vi "FlatToRichcif_channelcore_GetChannelsResponse.vi"(5 "OutputClusterType":T1, 11 "InputCluster":T6) -> (3 "OutputCluster":T1)   [LabVIEW 2021, in "CIFCoreChannel_client.lvlib"]
uses:
  CIFCoreChannel_client.lvlib
  cif_channelcore_GetChannelsResponse_Flat.ctl
  cif_management_common_Channels_Flat.ctl
  cif_management_common_Channel_Flat.ctl
  cif_management_common_ChannelDirection.ctl
  cif_management_common_ChannelPattern.ctl
  cif_channelcore_GetChannelsResponse.ctl
  cif_management_common_Channels.ctl
  cif_management_common_Channel.ctl
  FlatToRichcif_management_common_Channel.vi
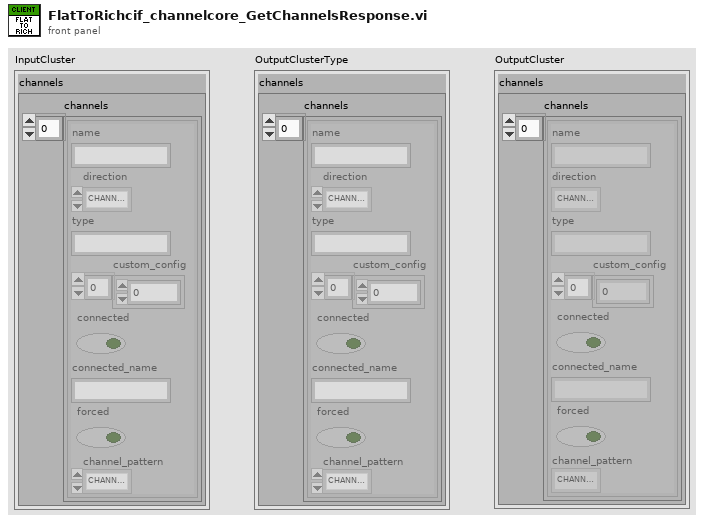
[diagram p1: front panel]
types:
  T1 = typedef "CIFCoreChannel_client.lvlib/cif_channelcore_GetChannelsResponse.ctl" = cluster{"channels":T2}
  T2 = typedef "CIFCoreChannel_client.lvlib/cif_management_common_Channels.ctl" = cluster{"channels":T3[]}
  T3 = typedef "CIFCoreChannel_client.lvlib/cif_management_common_Channel.ctl" = cluster{"name":string, "direction":T4, "type":string, "custom_config":u8[], "connected":bool, "connected_name":string, "forced":bool, "channel_pattern":T5}
  T4 = typedef "CIFCoreChannel_client.lvlib/cif_management_common_ChannelDirection.ctl" = enum32{"CHANNELDIRECTION_UNKNOWN", "CHANNELDIRECTION_PUBLISHER", "CHANNELDIRECTION_SUBSCRIBER"}
  T5 = typedef "CIFCoreChannel_client.lvlib/cif_management_common_ChannelPattern.ctl" = enum32{"CHANNELPATTERN_UNKNOWN", "CHANNELPATTERN_TAG", "CHANNELPATTERN_FIFO", "CHANNELPATTERN_MULTIFIFO", "CHANNELPATTERN_BACKPRESSUREFIFO"}
  T6 = typedef "CIFCoreChannel_client.lvlib/cif_channelcore_GetChannelsResponse_Flat.ctl" = cluster{"channels":T7}
  T7 = typedef "CIFCoreChannel_client.lvlib/cif_management_common_Channels_Flat.ctl" = cluster{"channels":T8[]}
  T8 = typedef "CIFCoreChannel_client.lvlib/cif_management_common_Channel_Flat.ctl" = cluster{"name":string, "direction":T4, "type":string, "custom_config":u8[], "connected":bool, "connected_name":string, "forced":bool, "channel_pattern":T5}
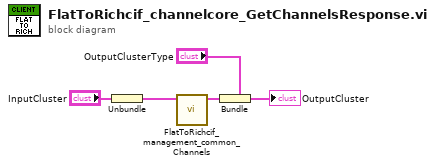
[diagram p0: block diagram]
diagram:
  n1 = Unbundle "Unbundle"("InputCluster") -> ("channels"=w2:T7)
  n2 = call "FlatToRichcif_management_common_Channels.vi"("InputCluster"=w2) -> ("OutputCluster"=w1:T2)  [unwired: 10 in]
  n3 = Bundle "Bundle"(cluster="OutputClusterType", "channels"=w1) -> (→"OutputCluster":T1)
